vi "z_rotmatrix.vi"(1 "z-angle":dbl format="%.2f") -> (0 "z-matrix":dbl[][](array[numeric]) format="%.2f")   [LabVIEW 2011]
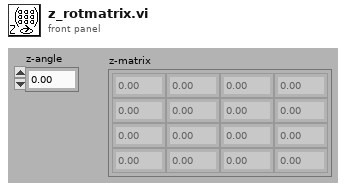
[diagram p1: front panel]
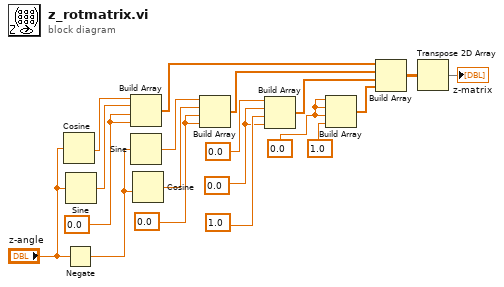
[diagram p0: block diagram]
diagram:
  w5 = 0.0
  w6 = 0.0
  w8 = 0.0
  w7 = 0.0
  n1 = Cosine(x="z-angle") -> (cos(x)=w16:dbl)
  n2 = Negate(x="z-angle") -> (-x=w10:dbl)
  n3 = Sine(x="z-angle") -> (sin(x)=w11:dbl)
  n4 = Build Array(w16, w11, w8, w8) -> (w17:dbl[])
  n5 = Sine(x=w10) -> (sin(x)=w15:dbl)
  n6 = Cosine(x=w10) -> (cos(x)=w9:dbl)
  n7 = Build Array(w15, w9, w7, w7) -> (w18:dbl[])
  n8 = Build Array(0.0, w6, 1.0, w6) -> (w19:dbl[])
  n9 = Build Array(w5, w5, w5, 1.0) -> (w3:dbl[])
  n10 = Build Array(w17, w18, w19, w3) -> (w2:dbl[][])
  n11 = Transpose 2D Array(2D array=w2) -> (transposed array=→"z-matrix":dbl[][])
